vi "Create Listener.vi"(8 "error in (no error)":errorcluster, 10 "Timeout ms (25000)":i32, 11 "TCP Server in":refnum<class "TCP Server.lvclass">) -> (0 "error out":errorcluster, 3 "TCP Server out":refnum<class "TCP Server.lvclass">)   [LabVIEW 2020, in "TCP Server.lvclass"]
uses:
  <vilib>/gpm_packages/@cs/Network-interface/Source/TCP Interface/TCP Server/TCP Server.lvclass
  <vilib>/gpm_packages/@cs/Network-interface/Source/TCP Interface/TCP Server/TCP Server.lvclass/TCP Server.ctl
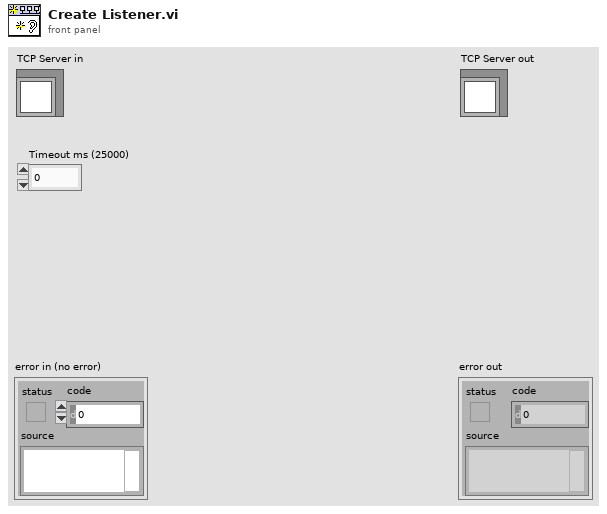
[diagram p1: front panel]
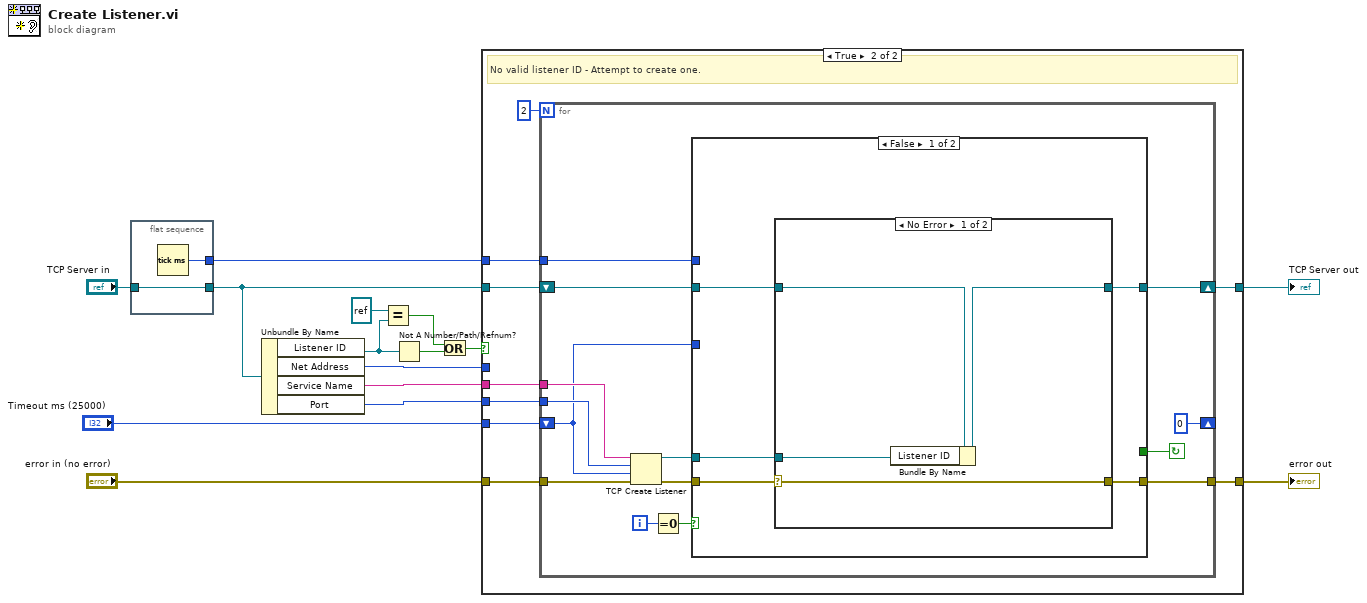
[diagram p0: block diagram]
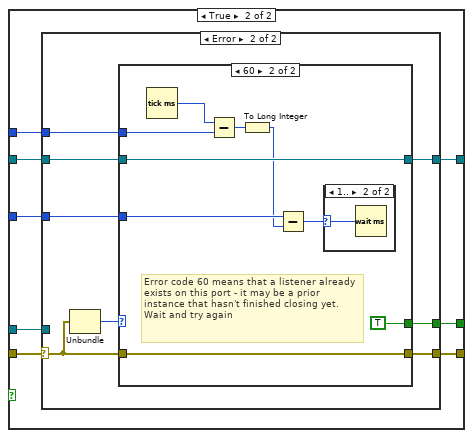
[diagram p4: hidden frame]
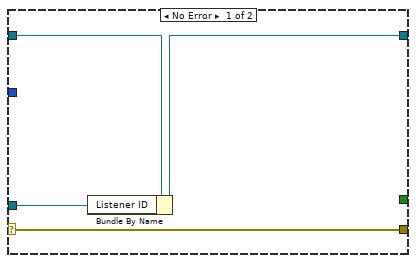
[diagram p5: hidden frame]
diagram:
  n1 = flat-sequence {
    tunnel: [w17] -> w3
    tunnel: "TCP Server in" -> [w17]
    tunnel: [w16] -> w1
    frame #0 {
      n2 = Tick Count (ms)() -> (millisecond timer value=w16:u32)
    }
  }
  n3 = Unbundle By Name(w3) -> ("Listener ID"=w8:refnum<k5>, "Net Address"=w12:u32, "Service Name"=w11:string, "Port"=w10:u16)
  n4 = Equal?(x=refnum<k5> refnum, y=w8) -> (x = y?=w6:bool)
  n5 = Not A Number/Path/Refnum?(number/path/refnum=w8) -> (NaN/Path/Refnum?=w9:bool)
  n6 = Or(x=w6, y=w9) -> (x .or. y?=w5:bool)
  n7 = case shown="True" w5 {
    tunnel: "error in (no error)" -> [w18 w28]
    tunnel: [w18 w23] -> w14
    tunnel: "Timeout ms (25000)" -> [_ w21]
    tunnel: w12 -> [_ _]
    tunnel: w11 -> [_ w27]
    tunnel: w10 -> [_ w26]
    tunnel: w3 -> [w19 w25]
    tunnel: [w19 w24] -> w4
    tunnel: w1 -> [_ w22]
    frame False {
      # "Already have a valid listener ID - don't create another"
    }
    frame True {
      # "No valid listener ID - Attempt to create one."
      n8 = for {
        N: 2 -> [_]
        tunnel: w27 -> [w41]
        tunnel: w26 -> [w40]
        tunnel: w22 -> [w34]
        shift-right: [w38] -> w24
        shift-left: w25 -> [w39]
        shift-right: [0 ("Timeout ms (25000)")] -> _
        shift-left: w21 -> [w33]
        tunnel: w28 -> [w42]
        tunnel: [w35] -> w23
        i -> [w30]
        stop <- w31 continue-if-true
        n9 = TCP Create Listener(8:w42, 9:w33, 10:w40, 11:w41) -> (0:w37:errorcluster, 3:w36:refnum<k5>)  [unwired: 1 in, 1 out]
        n10 = Equal To 0?(x=w30) -> (x = 0?=w29:bool)
        n11 = case shown="False" w29 {
          tunnel: w39 -> [w47 w61]
          tunnel: [w46 w60] -> w38
          tunnel: w37 -> [w45 w59]
          tunnel: w36 -> [w43 w58]
          tunnel: [w44 w57] -> w35
          tunnel: w34 -> [_ w56]
          tunnel: w33 -> [_ w55]
          tunnel: [_ w54] -> w31
          frame False {
            n12 = case shown="No Error" w45 {
              selector: w45 -> [w50 w52]
              tunnel: w47 -> [w51 w53]
              tunnel: [w49 w53] -> w46
              tunnel: [w50 w52] -> w44
              tunnel: w43 -> [w48 _]
              frame No Error {
                n13 = Bundle By Name(cluster=w51, "Listener ID"=w48) -> (w49:refnum<class "TCP Server.lvclass">)
              }
              frame Error {
              }
            }
          }
          frame True {
            n14 = case shown="Error" w59 {
              selector: w59 -> [w64 w73]
              tunnel: w61 -> [w65 w71]
              tunnel: [w63 w70] -> w60
              tunnel: w58 -> [w62 _]
              tunnel: [w64 w68] -> w57
              tunnel: w56 -> [_ w69]
              tunnel: w55 -> [_ w67]
              tunnel: [_ w66] -> w54
              frame No Error {
                n15 = Bundle By Name(cluster=w65, "Listener ID"=w62) -> (w63:refnum<class "TCP Server.lvclass">)
              }
              frame Error {
                n16 = Unbundle(w73) -> ("code"=w72:i32)  [unwired: 2 out]
                n17 = case shown="60" w72 {
                  tunnel: w73 -> [w74 w77]
                  tunnel: w71 -> [w75 w84]
                  tunnel: [w75 w84] -> w70
                  tunnel: w69 -> [_ w82]
                  tunnel: [w74 w77] -> w68
                  tunnel: w67 -> [_ w80]
                  tunnel: [_ TRUE] -> w66
                  frame 0, Default {
                  }
                  frame 60 {
                    # "Error code 60 means that a listener already exists on this port - it may be a prior instance that hasn't finished closing yet. Wait and try again"
                    n18 = Tick Count (ms)() -> (millisecond timer value=w83:u32)
                    n19 = Subtract(x=w83, y=w82) -> (x-y=w81:u32)
                    n20 = To Long Integer(number=w81) -> (32bit integer=w76:i32)
                    n21 = Subtract(x=w80, y=w76) -> (x-y=w79:i32)
                    n22 = case shown="1.." w79 {
                      selector: w79 -> [_ w85]
                      frame 0, Default {
                      }
                      frame 1.. {
                        n23 = Wait (ms)(milliseconds to wait=w85) -> ()  [unwired: 1 out]
                      }
                    }
                  }
                }
              }
            }
          }
        }
      }
    }
  }
  "error out" <- w14
  "TCP Server out" <- w4
